vi "After Launch Init Core.vi"(8 "error in (no error)":errorcluster, 10 "DelayInitialization?":bool, 11 "BNT_ULx-MCSV-Ctr2Freq in":refnum<class "BNT_ULx-MCSV-Ctr2Freq.lvclass">) -> (0 "error out":errorcluster, 3 "BNT_ULx-MCSV-Ctr2Freq out":refnum<class "BNT_ULx-MCSV-Ctr2Freq.lvclass">)   [LabVIEW 2020, in "BNT_ULx.lvlib" / "BNT_ULx-MCSV-Ctr2Freq.lvclass"]
doc: "Use <b>Pre Launch init.vi</b> method for sanity checks that are supposed to prevent the actor from launching if they fail. Use <B>this</B> method instead to initialize this actor when it has been activated. A corresponding high priority message will become dispatched before the <B>Actor Core.vi</b> is called.\n\n<b>Derived classed should call the parent methode first</b> and their own initialization code after.\n\nRefer also to the ongoing discussion at https://decibel.ni.com/content/message/57394#57394."
uses:
  BNT_ULx-MCSV-Ctr2Freq.lvclass
  BNT_ULx-MCSV-Ctr2Freq.lvclass/BNT_ULx-MCSV-Ctr2Freq.ctl
  BNT_ULx-MCSV/BNT_ULx-MCSV.lvclass
  CSPP_Core/Classes/CSPP_ProcessVariables/CSPP_ProcessVariables.lvlib
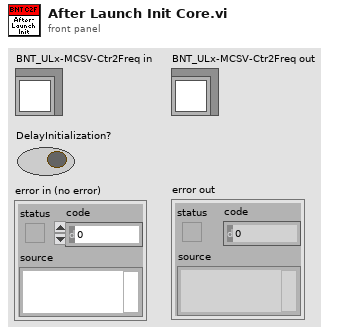
[diagram p1: front panel]
types:
  T1 = cluster{"Write Access":enum8{"Allowed", "Required", "None"}, "Read Access":enum8{"Allowed", "Required", "None"}}
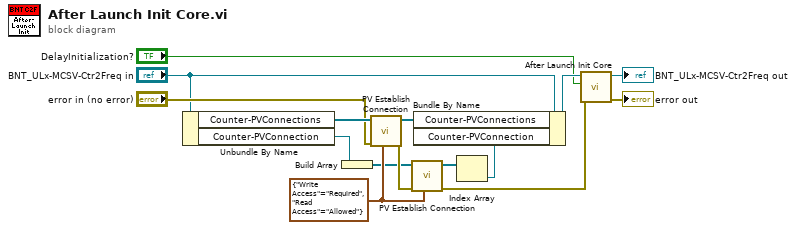
[diagram p0: block diagram]
diagram:
  w13 = T1 {"Write Access"=enum."Required", "Read Access"=enum."Allowed"} ("Access")
  n1 = Unbundle By Name("BNT_ULx-MCSV-Ctr2Freq in") -> ("Counter-PVConnections"=w8:refnum<class "PVConnection.lvclass">[], "Counter-PVConnection"=w11:refnum<class "PVConnection.lvclass">)
  n2 = Build Array(w11) -> (w10:refnum<class "PVConnection.lvclass">[])
  n3 = call "PV Establish Connection.vi"("Access (R/W allowed)"=w13, "Error In"="error in (no error)", "PVConnections in"=w8) -> ("Error Out"=w12:errorcluster, "PVConnections out"=w3:refnum<class "PVConnection.lvclass">[])  [unwired: 7 in]
  n4 = call "PV Establish Connection.vi"("Access (R/W allowed)"=w13, "Error In"=w12, "PVConnections in"=w10) -> ("Error Out"=w6:errorcluster, "PVConnections out"=w9:refnum<class "PVConnection.lvclass">[])  [unwired: 7 in]
  n5 = Index Array(array=w9) -> (element=w2:refnum<class "PVConnection.lvclass">)  [unwired: 1 in]
  n6 = Bundle By Name(cluster="BNT_ULx-MCSV-Ctr2Freq in", "Counter-PVConnections"=w3, "Counter-PVConnection"=w2) -> (w4:refnum<class "BNT_ULx-MCSV-Ctr2Freq.lvclass">)
  n7 = call-parent "After Launch Init Core.vi"("error in (no error)"=w6, "DelayInitialization?"="DelayInitialization?", "BNT_ULx-MCSV in"=w4) -> ("error out"=→"error out":errorcluster, "BNT_ULx-MCSV out"=→"BNT_ULx-MCSV-Ctr2Freq out":refnum<class "BNT_ULx-MCSV-Ctr2Freq.lvclass">)  [unwired: 7 in]
